vi "Top Level State Machine.vi"() -> ()   [LabVIEW 2014]
uses:
  Scripting States.ctl
  System.Windows.Forms
  Initialization Scripting/Initialization and IO Node Scripting.lvlib
panel:
  in  "Number of Channels per Device":i32[][](array[numeric])
  in  "Number of SPI Devices on Bus":i32[](array[numeric])
  in  "Number of SPI Buses":i32=1
  in  "Enable":bool[](array[boolean])=[TRUE, FALSE, FALSE, FALSE, TRUE, FALSE, TRUE, TRUE, TRUE]
  in  "List of Enable Lines":string[](array[string])=["sbRIO-9651 Socket\\PMOD1_Pin3_enable", "sbRIO-9651 Socket\\PMOD1_Pin4_enable"]
  in  "List of IO Names":string[](array[string])=["Port0/DIO0", "Port0/DIO5", "Port0/DIO6"]
  in  "Path to Test VI to Place (IO Nodes and SPI Engine Placed on Block Diagram)":path=path "C:/Users/mpool/Desktop/test/TestVI.vi"
  in  "Path to Test Project":path=path "C:/Users/lvadmin/Desktop/Scripting/Test/Test.lvproj"
  in  "Destination Path":path=path "C:/Users/kvemishe/Downloads/TestScript"
  in  "Golden Template Source Path":path=path "C:/Users/kvemishe/Desktop/IONode"
  out "Elapsed Time":dbl format="%<%H:%M:%S>t"
  in  "ProgressBar":refnum<k24>(container)
  in  "?":T1
  out "Status Log":string
  out "Progress Bar":u8(slide) scale=0.0..9.0
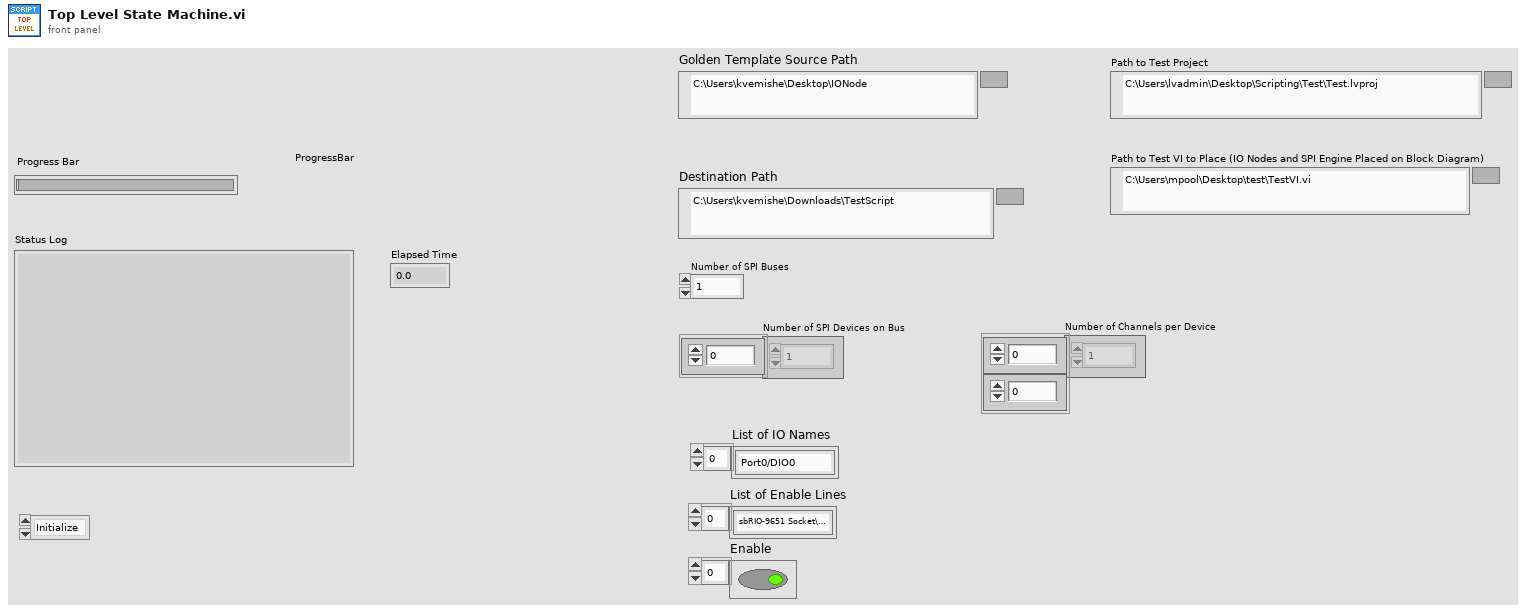
[diagram p1: front panel]
types:
  T1 = typedef "Scripting States.ctl" = enum16{"Initialize", "Modify Dequeue Commands", "Modify Enqueue Data", "Create Project FIFOs", "Create and Place IO Nodes", "Populate FIFO Names in Engine", "Modify I/O Pin Names", "Modify I/O Pin Enable", "Place SPI Engine", "End"}
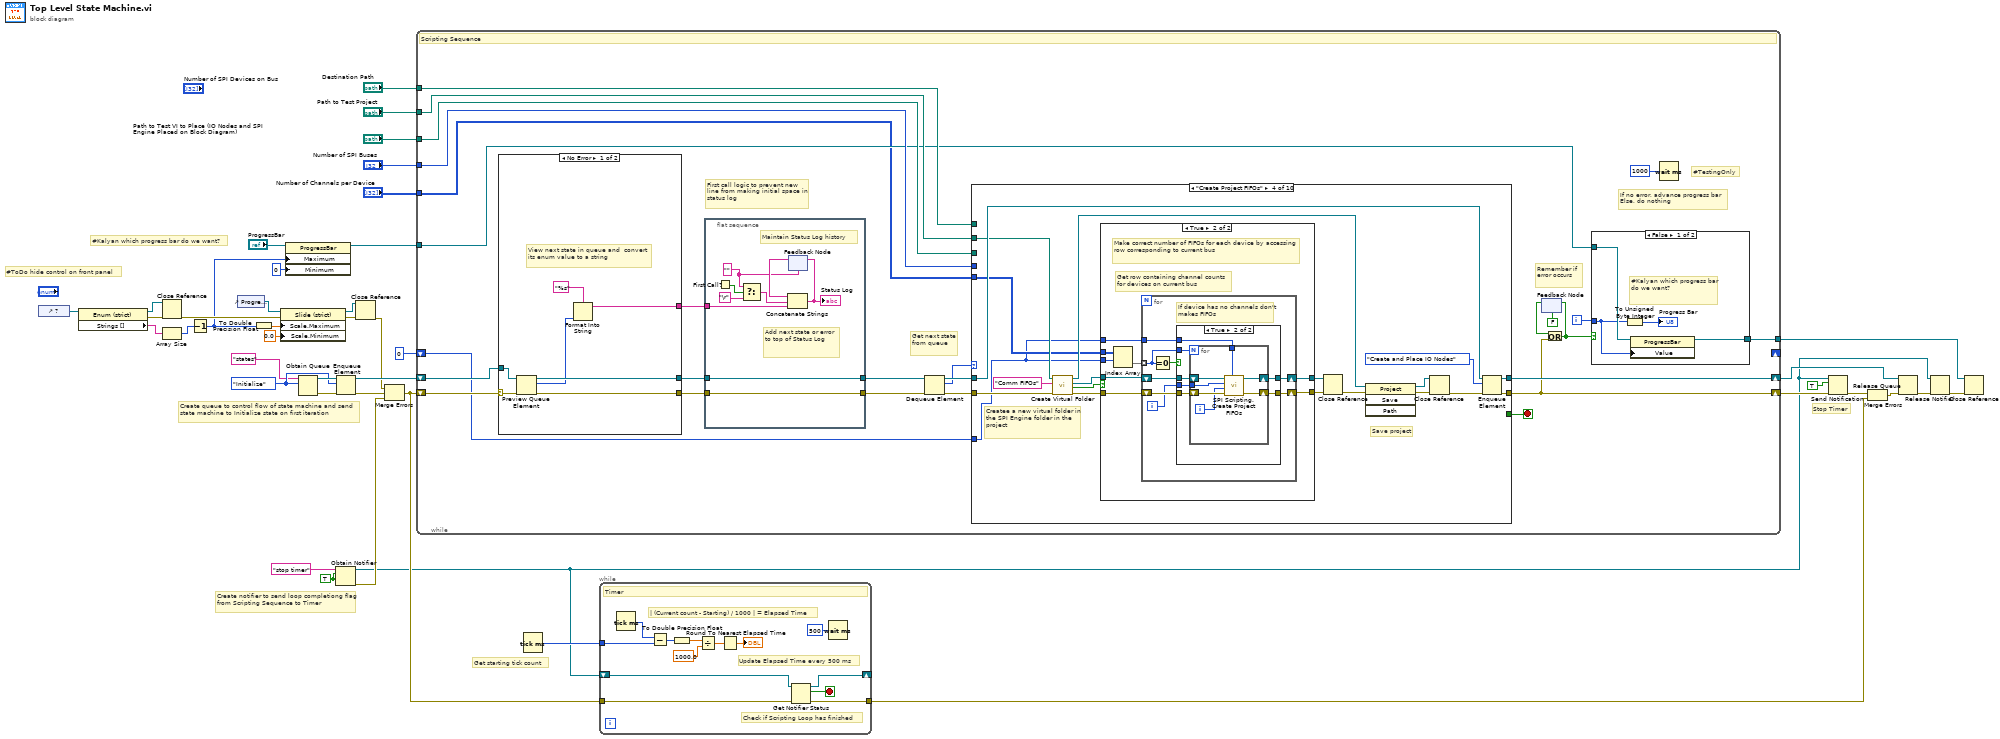
[diagram p0: block diagram]
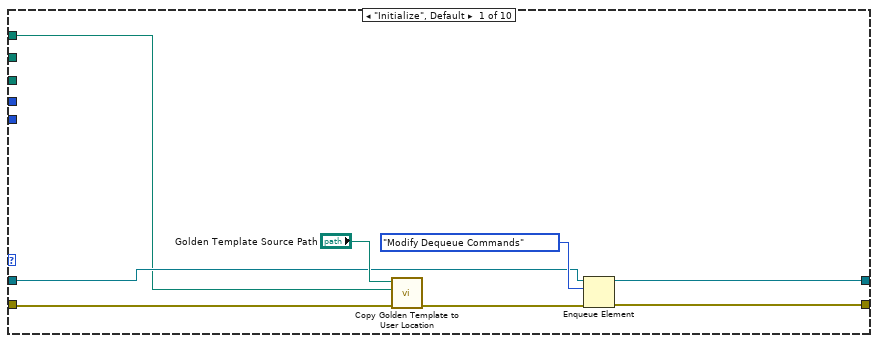
[diagram p3: hidden frame]
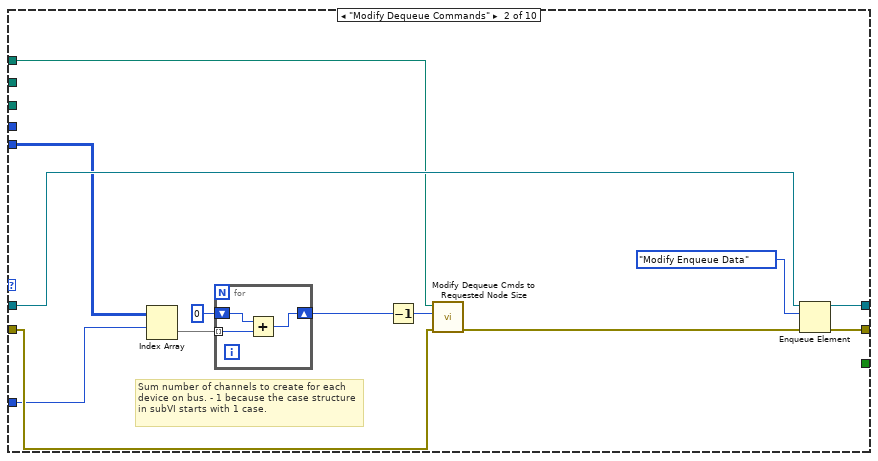
[diagram p4: hidden frame]
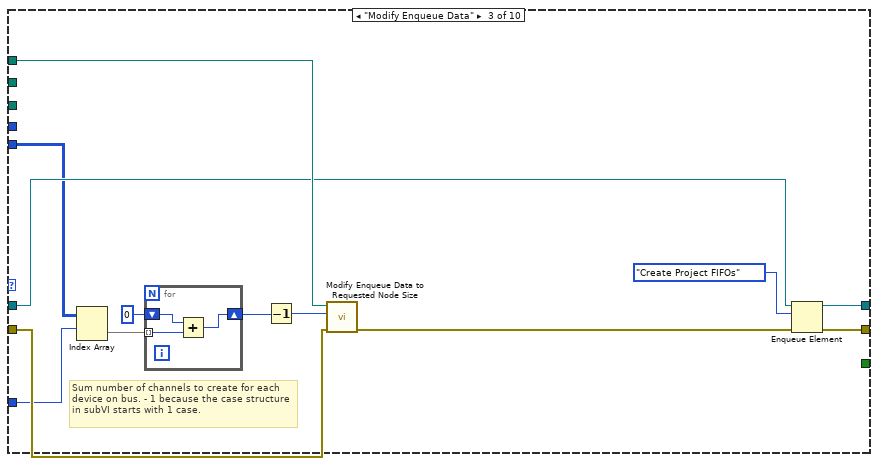
[diagram p5: hidden frame]
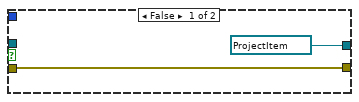
[diagram p6: hidden frame]
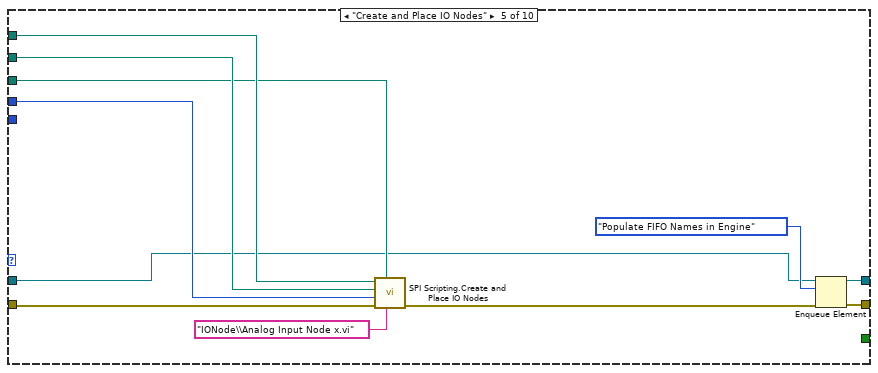
[diagram p8: hidden frame]
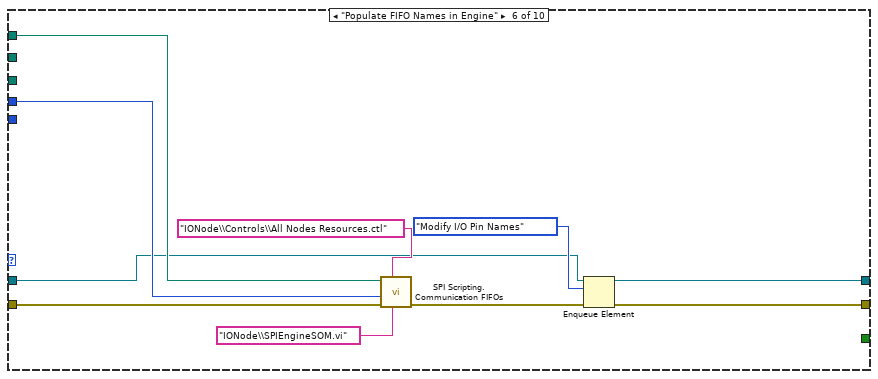
[diagram p9: hidden frame]
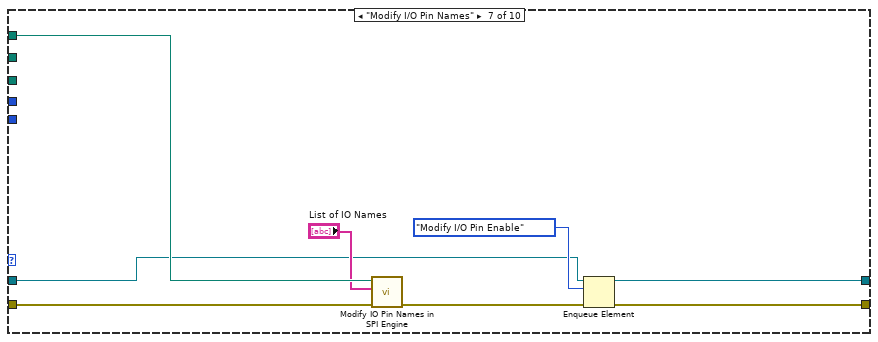
[diagram p10: hidden frame]
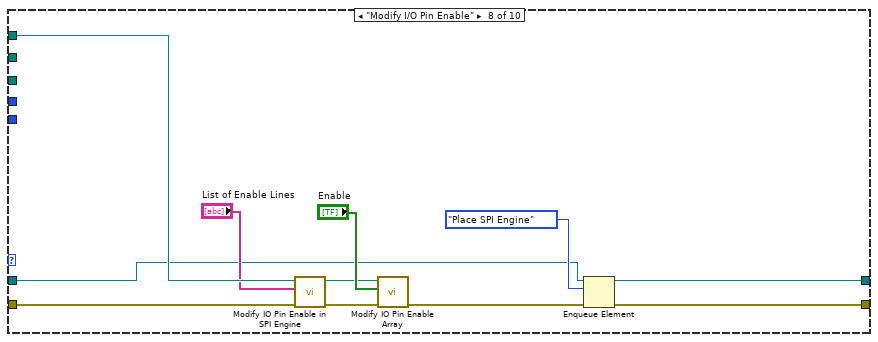
[diagram p11: hidden frame]
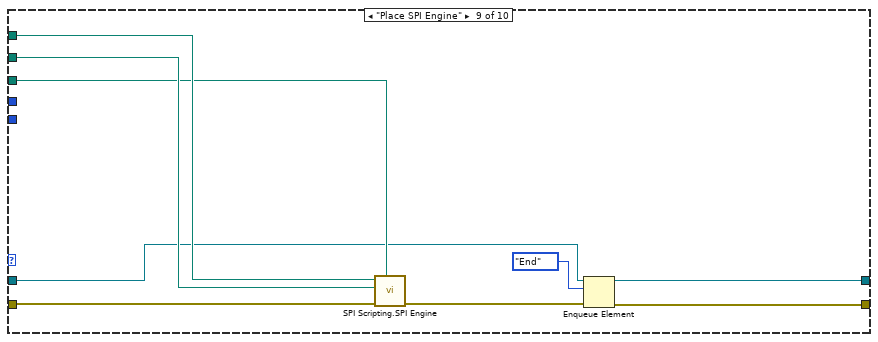
[diagram p12: hidden frame]
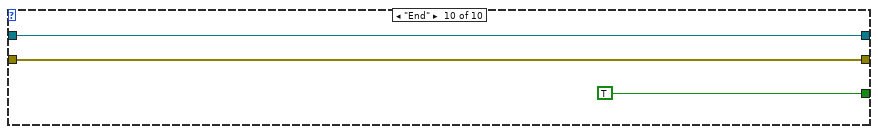
[diagram p13: hidden frame]
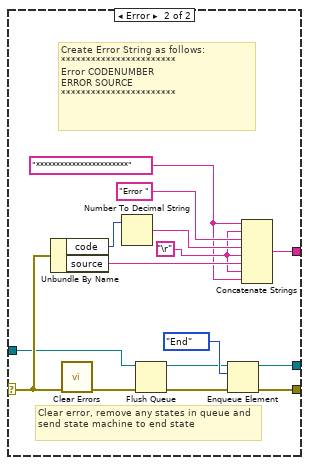
[diagram p14: hidden frame]
diagram:
  w20 = TRUE ("create if not found? (T)")
  w37 = Scripting_States."Initialize"
  # "#ToDo hide control on front panel"
  # "Get starting tick count"
  # "Stop Timer"
  # "Create notifier to send loop completiong flag from Scripting Sequence to Timer"
  # "Create queue to control flow of state machine and send state machine to Initialize state on first iteration"
  # "#Kalyan which progress bar do we want?"
  n1 = control-ref of="?"() -> (w43:refnum<vi>)
  n2 = property on="Property Node" class="Enum (strict)"(reference=w43) -> (reference out=w30:refnum<vi>, error out=w31:errorcluster, "Strings []"=w42:string[])  [unwired: 1 in]
  n3 = Close Reference(reference=w30, error in (no error)=w31) -> (error out=w28:errorcluster)
  n4 = Array Size(array=w42) -> (size(s)=w27:i32)
  n5 = Decrement(x=w27) -> (x-1=w25:i32)
  n6 = control-ref of="Progress Bar"() -> (w41:refnum<vi>)
  n7 = To Double Precision Float(number=w25) -> (double precision float=w40:dbl)
  n8 = property on="Property Node" class="Slide (strict)"(reference=w41, error in=w28, "Scale.Maximum"=w40, "Scale.Minimum"=0.0 ("Scale.Range:Minimum")) -> (reference out=w32:refnum<vi>, error out=w33:errorcluster)
  n9 = property class="ProgressBar"(reference="ProgressBar", "Maximum"=w25, "Minimum"=0) -> (reference out=w15:refnum<k24>)  [unwired: 1 in, 1 out]
  n10 = Obtain Queue(name (unnamed)="states", element data type=w37) -> (queue out=w38:refnum<queue>, error out=w39:errorcluster)  [unwired: 3 in, 1 out]
  n11 = Obtain Notifier(name (unnamed)="stop timer", notification data type=w20, create if not found? (T)=w20) -> (notifier out=w8:refnum<notifier>, error out=w22:errorcluster)  [unwired: 1 in, 1 out]
  n12 = Enqueue Element(queue=w38, element=w37, error in (no error)=w39) -> (queue out=w35:refnum<queue>, error out=w34:errorcluster)  [unwired: 1 in, 1 out]
  n13 = Close Reference(reference=w32, error in (no error)=w33) -> (error out=w29:errorcluster)
  n14 = Merge Errors(w29, w34, w22) -> (w21:errorcluster)
  n15 = while {
    shift-right: [w63] -> w10
    shift-left: w21 -> [w69]
    shift-right: [w64] -> w9
    shift-left: w35 -> [w68]
    tunnel: [w53] -> w16
    tunnel: w15 -> [w46]
    tunnel: "Destination Path" -> [w52]
    tunnel: "Path to Test Project" -> [w50]
    tunnel: "Path to Test VI to Place (IO Nodes and SPI Engine Placed on Block Diagram)" -> [w51]
    tunnel: "Number of SPI Buses" -> [w49]
    tunnel: "Number of Channels per Device" -> [w45]
    shift-right: _ -> [_]
    shift-left: 0 ("Number of SPI Buses") -> [w44]
    i -> [w48]
    stop <- w47 stop-if-true
    # "First call logic to prevent new line from making initial space in status log"
    # "If no error, advance progress bar\nElse, do nothing"
    # "Remember if error occurs"
    # "Get next state from queue"
    # "#TestingOnly"
    # "Scripting Sequence"
    n16 = case shown="No Error" w69 {
      selector: w69 -> [w235 w245]
      tunnel: [w229 w247] -> w58
      tunnel: w68 -> [w234 w240]
      tunnel: [w232 w244] -> w57
      tunnel: [w233 w243] -> w55
      frame No Error {
        # "View next state in queue and  convert its enum value to a string"
        n17 = Preview Queue Element(queue=w234, error in (no error)=w235) -> (queue out=w233:refnum<queue>, element=w230:T1, error out=w232:errorcluster)  [unwired: 1 in, 1 out]
        n18 = Format Into String "Format Into String"(format string="%s", w230) -> (resulting string=w229:string)  [unwired: 2 in, 1 out]
      }
      frame Error {
        w236 = "***********************" ("string")
        w237 = "\r"
        # "Create Error String as follows:\n***********************\nError CODENUMBER\nERROR SOURCE\n***********************"
        # "Clear error, remove any states in queue and send state machine to end state"
        n19 = Unbundle By Name(w245) -> ("code"=w248:i32, "source"=w250:string)
        n20 = call <vilib>:"Clear Errors.vi"("error in (no error)"=w245) -> ("error out"=w242:errorcluster)  [unwired: 5 in, 1 out]
        n21 = Number To Decimal String(number=w248) -> (decimal integer string=w249:string)  [unwired: 1 in]
        n22 = Flush Queue(queue=w240, error in (no error)=w242) -> (queue out=w239:refnum<queue>, error out=w241:errorcluster)  [unwired: 1 out]
        n23 = Enqueue Element(queue=w239, element=Scripting_States."End", error in (no error)=w241) -> (queue out=w243:refnum<queue>, error out=w244:errorcluster)  [unwired: 1 in, 1 out]
        n24 = Concatenate Strings(w236, w237, "Error " ("string"), w249, w237, w250, w237, w236) -> (w247:string)
      }
    }
    n25 = flat-sequence {
      tunnel: w58 -> [w74]
      tunnel: w57 -> [w77]
      tunnel: [w77] -> w56
      tunnel: [w76] -> w54
      tunnel: w55 -> [w76]
      frame #0 {
        w70 = ""
        # "Add next state or error to top of Status Log"
        # "Maintain Status Log history"
        n26 = First Call?() -> (First Call?: T/F=w71:bool)
        n27 = Select(t=w70, s=w71, f="\r") -> (s? t:f=w72:string)
        n28 = feedback #1(w70) -> (w75:string)
        n29 = Concatenate Strings(w75, w72, w74) -> (w78:string)
        "Status Log" <- w78
        n30 = feedback-in #1(w78) -> ()
      }
    }
    n31 = Dequeue Element(queue=w54, error in (no error)=w56) -> (queue out=w66:refnum<queue>, element=w65:T1, error out=w67:errorcluster)  [unwired: 1 in, 1 out]
    n32 = case shown="\"Create Project FIFOs\"" w65 {
      tunnel: [w90 w103 w119 w141 w186 w196 w204 w215 w224 w226] -> w63
      tunnel: [w91 w104 w120 w142 w187 w197 w205 w216 w225 w227] -> w64
      tunnel: [_ _ _ _ _ _ _ _ _ TRUE] -> w47
      tunnel: w67 -> [w87 w96 w109 w137 w184 w194 w202 w213 w222 w226]
      tunnel: w66 -> [w85 w101 w116 w139 w178 w189 w198 w206 w217 w227]
      tunnel: w52 -> [w84 w99 w117 _ w182 w193 w201 w210 w220 _]
      tunnel: w50 -> [_ _ _ w136 w181 _ _ _ w219 _]
      tunnel: w51 -> [_ _ _ _ w180 _ _ _ w218 _]
      tunnel: w49 -> [_ _ _ _ w179 w192 _ _ _ _]
      tunnel: w45 -> [_ w97 w110 w125 _ _ _ _ _ _]
      tunnel: w44 -> [_ w92 w108 w124 _ _ _ _ _ _]
      frame "Initialize", Default {
        n33 = call "Copy Golden Template to User Location.vi"("Error In"=w87, "Current Engine Path"=w84, "Golden Template Path"="Golden Template Source Path") -> ("error out"=w86:errorcluster)  [unwired: 8 in]
        n34 = Enqueue Element(queue=w85, element=Scripting_States."Modify Dequeue Commands", error in (no error)=w86) -> (queue out=w91:refnum<queue>, error out=w90:errorcluster)  [unwired: 1 in, 1 out]
      }
      frame "Modify Dequeue Commands" {
        # "Sum number of channels to create for each device on bus. - 1 because the case structure in subVI starts with 1 case."
        n35 = Index Array(array=w97, index (row)=w92) -> (element=w95:i32[])  [unwired: 1 in]
        n36 = for {
          tunnel: w95 -> [w107] mode=indexing
          shift-right: [w105] -> w93
          shift-left: 0 -> [w106]
          n37 = Add(x=w106, y=w107) -> (x+y=w105:i32)
        }
        n38 = Decrement(x=w93) -> (x-1=w98:i32)
        n39 = call "Modify Dequeue Cmds to Requested Node Size.vi"("Error In"=w96, "NumCasesToAdd"=w98, "Source Root Path"=w99) -> ("Error Out"=w100:errorcluster)  [unwired: 6 in, 2 out]
        n40 = Enqueue Element(queue=w101, element=Scripting_States."Modify Enqueue Data", error in (no error)=w100) -> (queue out=w104:refnum<queue>, error out=w103:errorcluster)  [unwired: 1 in, 1 out]
      }
      frame "Modify Enqueue Data" {
        # "Sum number of channels to create for each device on bus. - 1 because the case structure in subVI starts with 1 case."
        n41 = Index Array(array=w110, index (row)=w108) -> (element=w113:i32[])  [unwired: 1 in]
        n42 = for {
          tunnel: w113 -> [w123] mode=indexing
          shift-right: [w121] -> w111
          shift-left: 0 -> [w122]
          n43 = Add(x=w122, y=w123) -> (x+y=w121:i32)
        }
        n44 = Decrement(x=w111) -> (x-1=w114:i32)
        n45 = call "Modify Enqueue Data to Requested Node Size.vi"("Error In"=w109, "NumCasesToAdd"=w114, "Source Root Path"=w117) -> ("error out"=w115:errorcluster)  [unwired: 6 in, 2 out]
        n46 = Enqueue Element(queue=w116, element=Scripting_States."Create Project FIFOs", error in (no error)=w115) -> (queue out=w120:refnum<queue>, error out=w119:errorcluster)  [unwired: 1 in, 1 out]
      }
      frame "Create Project FIFOs" {
        # "Save project"
        # "Createe a new virtual folder in the SPI Engine folder in the project"
        n47 = call "Create Virtual Folder.vi"("error in"=w137, "Virtual Folder Name"="Comm FIFOs", "Path to Project"=w136) -> ("error out"=w129:errorcluster, "FPGA Target Found"=w127:bool, "New Virtual Folder"=w126:refnum<vi>, "Project:Open"=w130:refnum<vi>)  [unwired: 5 in]
        n48 = case shown="True" w127 {
          tunnel: [w144 w152] -> w131
          tunnel: w129 -> [w144 w151]
          tunnel: [refnum<vi> refnum ("Comm FIFOs Virtual Folder") w150] -> w128
          tunnel: w126 -> [_ w149]
          tunnel: w125 -> [_ w148]
          tunnel: w124 -> [_ w147]
          tunnel: w124 -> [_ w145]
          frame False {
          }
          frame True {
            # "Make correct number of FIFOs for each device by accessing row corresponding to current bus"
            # "Get row containing channel counts for devices on current bus"
            n49 = Index Array(array=w148, index (row)=w147) -> (element=w146:i32[])  [unwired: 1 in]
            n50 = for {
              shift-right: [w160] -> w152
              shift-left: w151 -> [w159]
              tunnel: w146 -> [w154] mode=indexing
              shift-right: [w158] -> w150
              shift-left: w149 -> [w157]
              tunnel: w145 -> [w153]
              i -> [w155]
              # "If device has no channels don't makes FIFOs"
              n51 = Equal To 0?(x=w154) -> (x = 0?=w156:bool)
              n52 = case shown="True" w156 {
                tunnel: [w162 w169] -> w160
                tunnel: w159 -> [w162 w168]
                tunnel: [w161 w167] -> w158
                tunnel: w157 -> [w161 w166]
                tunnel: w155 -> [_ w165]
                tunnel: w154 -> [_ w164]
                tunnel: w153 -> [_ w163]
                frame False {
                }
                frame True {
                  n53 = for {
                    N: w164 -> [_]
                    shift-right: [w176] -> w169
                    shift-left: w168 -> [w175]
                    shift-right: [w174] -> w167
                    shift-left: w166 -> [w173]
                    tunnel: w165 -> [w171]
                    tunnel: w163 -> [w170]
                    i -> [w172]
                    n54 = call "SPI Scripting.Create Project FIFOs.vi"("Bus Number"=w170, "error in"=w175, "Channel Number"=w172, "Device Number"=w171, "New Virtual Folder"=w173) -> ("error out"=w176:errorcluster, "Comm FIFOs Virtual Folder"=w174:refnum<vi>)  [unwired: 5 in]
                  }
                }
              }
            }
          }
        }
        n55 = Close Reference(reference=w128, error in (no error)=w131) -> (error out=w135:errorcluster)
        n56 = invoke class="Project" method="Save"(reference=w130, error in=w135) -> (reference out=w133:refnum<vi>, error out=w134:errorcluster)  [unwired: 2 in, 2 out]
        n57 = Close Reference(reference=w133, error in (no error)=w134) -> (error out=w132:errorcluster)
        n58 = Enqueue Element(queue=w139, element=Scripting_States."Create and Place IO Nodes", error in (no error)=w132) -> (queue out=w142:refnum<queue>, error out=w141:errorcluster)  [unwired: 1 in, 1 out]
      }
      frame "Create and Place IO Nodes" {
        n59 = call "SPI Scripting.Create and Place IO Nodes.vi"("Path to Analog Node"="IONode\\Analog Input Node x.vi" ("Path to SOM Engine"), "Path to Place IO Node"=w180, "error in"=w184, "Number of SPI Devices on Bus"=w179, "Path to Project"=w181, "Path to IO Node"=w182) -> ("error out"=w183:errorcluster)  [unwired: 3 in, 2 out]
        n60 = Enqueue Element(queue=w178, element=Scripting_States."Populate FIFO Names in Engine", error in (no error)=w183) -> (queue out=w187:refnum<queue>, error out=w186:errorcluster)  [unwired: 1 in, 1 out]
      }
      frame "Populate FIFO Names in Engine" {
        n61 = call "SPI Scripting.Communication FIFOs.vi"("Path to SOM Engine"="IONode\\SPIEngineSOM.vi", "Path to All Nodes Resources"="IONode\\Controls\\All Nodes Resources.ctl", "error in"=w194, "Number of SPI Devices on Bus"=w192, "Path to IO Node"=w193) -> ("error out"=w188:errorcluster)  [unwired: 4 in, 2 out]
        n62 = Enqueue Element(queue=w189, element=Scripting_States."Modify I/O Pin Names", error in (no error)=w188) -> (queue out=w197:refnum<queue>, error out=w196:errorcluster)  [unwired: 1 in, 1 out]
      }
      frame "Modify I/O Pin Names" {
        n63 = call "Modify IO Pin Names in SPI Engine.vi"("Error In"=w202, "List of IO Names"="List of IO Names", "Source Root Path"=w201) -> ("Error Out"=w200:errorcluster)  [unwired: 6 in, 2 out]
        n64 = Enqueue Element(queue=w198, element=Scripting_States."Modify I/O Pin Enable", error in (no error)=w200) -> (queue out=w205:refnum<queue>, error out=w204:errorcluster)  [unwired: 1 in, 1 out]
      }
      frame "Modify I/O Pin Enable" {
        n65 = call "Modify IO Pin Enable in SPI Engine.vi"("Error In"=w213, "List of Enable Lines"="List of Enable Lines", "Source Root Path"=w210) -> ("Error Out"=w212:errorcluster, "Source Root Path Out"=w207:path)  [unwired: 6 in, 1 out]
        n66 = call "Modify IO Pin Enable Array.vi"("Error In"=w212, "Enable"="Enable", "Source Root Path"=w207) -> ("Error Out"=w211:errorcluster)  [unwired: 6 in, 2 out]
        n67 = Enqueue Element(queue=w206, element=Scripting_States."Place SPI Engine", error in (no error)=w211) -> (queue out=w216:refnum<queue>, error out=w215:errorcluster)  [unwired: 1 in, 1 out]
      }
      frame "Place SPI Engine" {
        n68 = call "SPI Scripting.SPI Engine.vi"("Path to Place SPI Engine"=w218, "error in"=w222, "Path to Project"=w219, "Path to IO Node"=w220) -> ("error out"=w221:errorcluster)  [unwired: 6 in, 1 out]
        n69 = Enqueue Element(queue=w217, element=Scripting_States."End", error in (no error)=w221) -> (queue out=w225:refnum<queue>, error out=w224:errorcluster)  [unwired: 1 in, 1 out]
      }
      frame "End" {
      }
    }
    n70 = feedback #2(FALSE) -> (w62:bool)
    n71 = Or(x=w62, y=w63) -> (x .or. y?=w60:bool)
    n72 = feedback-in #2(w60) -> ()
    n73 = case shown="False" w60 {
      tunnel: w48 -> [w80 _]
      tunnel: [w82 w83] -> w53
      tunnel: w46 -> [w81 w83]
      frame False {
        # "#Kalyan which progress bar do we want?"
        n74 = To Unsigned Byte Integer(number=w80) -> (unsigned 8bit integer=→"Progress Bar":u8)
        n75 = property class="ProgressBar"(reference=w81, "Value"=w80) -> (reference out=w82:refnum<k24>)  [unwired: 1 in, 1 out]
      }
      frame True {
      }
    }
    n76 = Wait (ms)(milliseconds to wait=u32 1000) -> ()  [unwired: 1 out]
  }
  n77 = Tick Count (ms)() -> (millisecond timer value=w23:u32)
  n78 = while {
    tunnel: w23 -> [w262]
    tunnel: w21 -> [w254]
    shift-right: [w252] -> _
    shift-left: w8 -> [w255]
    tunnel: [w251] -> w13
    stop <- w253 stop-if-true
    # "Update Elapsed Time every 500 ms"
    # "| (Current count - Starting) / 1000 | = Elapsed Time"
    # "Check if Scripting Loop has finished"
    # "Timer"
    n79 = Tick Count (ms)() -> (millisecond timer value=w263:u32)
    n80 = Subtract(x=w263, y=w262) -> (x-y=w261:u32)
    n81 = To Double Precision Float(number=w261) -> (double precision float=w260:dbl)
    n82 = Divide(x=w260, y=1000.0) -> (x/y=w258:dbl)
    n83 = Round To Nearest(number=w258) -> (nearest integer value=→"Elapsed Time":dbl)
    n84 = Get Notifier Status(notifier=w255, error in (no error)=w254) -> (notifier out=w252:refnum<notifier>, current notification=w253:bool, error out=w251:errorcluster)  [unwired: 2 out]
    n85 = Wait (ms)(milliseconds to wait=u32 500) -> ()  [unwired: 1 out]
  }
  n86 = Send Notification(notification=TRUE, notifier=w8, error in (no error)=w10) -> (error out=w11:errorcluster)  [unwired: 1 out]
  n87 = Merge Errors(w11, w13) -> (w14:errorcluster)
  n88 = Release Queue(queue=w9, error in (no error)=w14) -> (error out=w18:errorcluster)  [unwired: 1 in, 2 out]
  n89 = Release Notifier(notifier=w8, error in (no error)=w18) -> (error out=w17:errorcluster)  [unwired: 1 in, 2 out]
  n90 = Close Reference(reference=w16, error in (no error)=w17) -> ()  [unwired: 1 out]
